vi "addEdge.vi"(0 "reference":refnum<class "NoteNode.lvclass">, 1 "egde":refnum<class "AbstractEdge.lvclass">, 2 "p1":T1 {"y" format="%.2f"; "x" format="%.2f"}, 3 "p2":T1 {"y" format="%.2f"; "x" format="%.2f"}, 5 "error in (no error)":errorcluster) -> (14 "reference out":refnum<class "NoteNode.lvclass">, 15 "edgeHasEndNode":bool, 19 "error out":errorcluster)   [LabVIEW 2012, in "NoteNode.lvclass"]
doc: "public boolean addEdge(Edge e, Point2D p1, Point2D p2)"
uses:
  <resource>/Framework/Providers/Open_GDS/UML/NoteNode_class/NoteNode.lvclass
  <resource>/Framework/Providers/Open_GDS/UML/AbstractEdge_class/AbstractEdge.lvclass
  <resource>/Framework/Providers/Open_GDS/UML/General/Point/Point Point2D.ctl
  <resource>/Framework/Providers/Open_GDS/UML/RectangularNode_class/RectangularNode.lvclass
  <resource>/Framework/Providers/Open_GDS/UML/PointNode_class/PointNode.lvclass
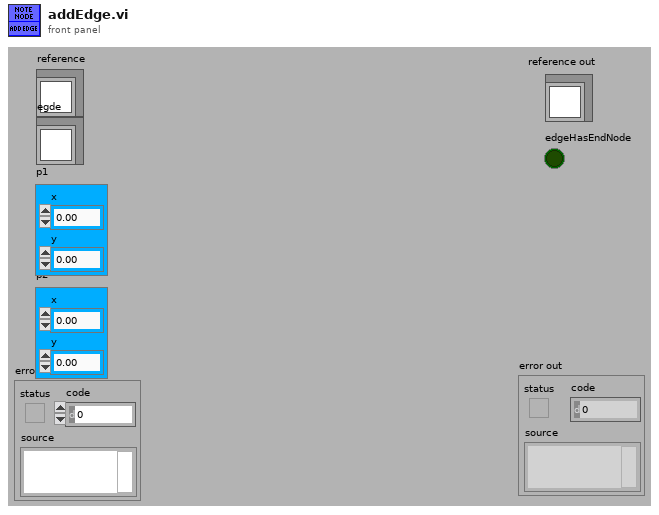
[diagram p1: front panel]
types:
  T1 = typedef "Point Point2D.ctl" = cluster{"x":dbl, "y":dbl}
  T2 = typedef "NoteNode.lvclass/ObjectAttributes.ctl" = cluster{"Base class":T3, "DEFAULT_WIDTH":i32, "DEFAULT_HEIGHT":i32, "DEFAULT_COLOR":u32, "FOLD_X":i32, "FOLD_Y":i32, "color":u32, "text":refnum<class "MultiLineString.lvclass">, "pointNodes":refnum<class "AbstractNode.lvclass">[]}
  T3 = typedef "RectangularNode.lvclass/ObjectAttributes.ctl" = cluster{"Base class":T4, "bounds":T5}
  T4 = typedef "AbstractNode.lvclass/ObjectAttributes.ctl" = cluster{"parent":refnum<class "AbstractNode.lvclass">, "children":refnum<class "AbstractNode.lvclass">[], "Hidden":bool}
  T5 = typedef "Rectangle Rectangle2D.ctl" = cluster{"x":dbl, "y":dbl, "width":dbl, "height":dbl}
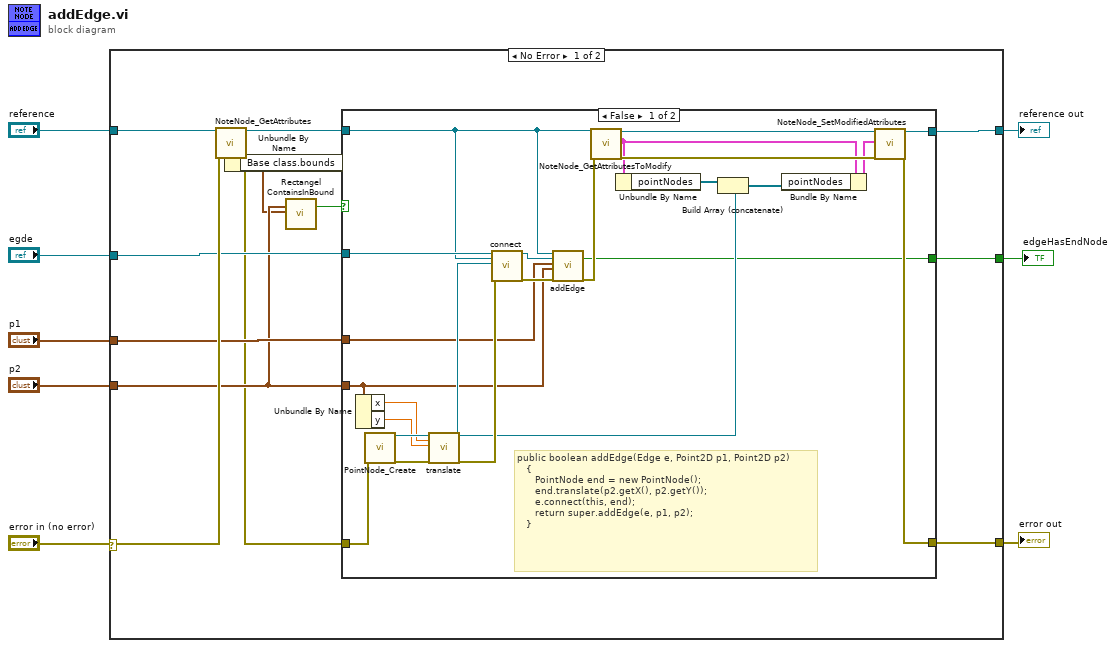
[diagram p0: block diagram]
diagram:
  n1 = case shown="No Error" "error in (no error)" {
    selector: "error in (no error)" -> [w18 w47]
    tunnel: "reference" -> [w21 w48]
    tunnel: [w20 w47] -> w7
    tunnel: [w19 w48] -> w6
    tunnel: "egde" -> [w17 _]
    tunnel: "p1" -> [w16 _]
    tunnel: "p2" -> [w15 _]
    tunnel: [w9 _] -> w1
    frame No Error {
      n2 = call <resource>:"NoteNode_GetAttributes.vi"("reference in"=w21, "error in (no error)"=w18) -> ("reference out"=w14:refnum<class "NoteNode.lvclass">, "Attributes"=w12:T2, "error out"=w13:errorcluster)  [unwired: 15 out]
      n3 = Unbundle By Name(w12) -> ("Base class.bounds"=w11:T5)
      n4 = call <resource>:"Rectangel ContainsInBound.vi"("point2D"=w15, "bounds"=w11) -> ("contains"=w10:bool)  [unwired: 2 in, 15 out]
      n5 = case shown="False" w10 {
        tunnel: w17 -> [w44 _]
        tunnel: w16 -> [w25 _]
        tunnel: [w36 w46] -> w19
        tunnel: [w35 w45] -> w20
        tunnel: w14 -> [w28 w46]
        tunnel: w13 -> [w29 w45]
        tunnel: w15 -> [w24 _]
        tunnel: [w22 _] -> w9
        frame False {
          # "public boolean addEdge(Edge e, Point2D p1, Point2D p2)\n   {\n      PointNode end = new PointNode();\n      end.translate(p2.getX(), p2.getY());\n      e.connect(this, end);\n      return super.addEdge(e, p1, p2);\n   }"
          n6 = Unbundle By Name(w24) -> ("x"=w41:dbl, "y"=w40:dbl)
          n7 = call <resource>:"PointNode_Create.vi"("error in (no error)"=w29) -> ("reference out"=w43:refnum<class "PointNode.lvclass">, "error out"=w42:errorcluster)  [unwired: 2 in, 15 out]
          n8 = call-dynamic "translate.vi"("reference"=w43, "dx"=w41, "dy"=w40, "error in (no error)"=w42) -> ("reference out"=w30:refnum<class "PointNode.lvclass">, "error out"=w39:errorcluster)  [unwired: 14 in]
          n9 = call-dynamic "connect.vi"("reference"=w44, "startNode"=w28, "endNode"=w30, "error in (no error)"=w39) -> ("reference out"=w26:refnum<class "AbstractEdge.lvclass">, "error out"=w27:errorcluster)  [unwired: 14 in]
          n10 = call-parent "addEdge.vi"("reference"=w28, "egde"=w26, "p1"=w25, "p2"=w24, "error in (no error)"=w27) -> ("edgeHasEndNode"=w22:bool, "error out"=w23:errorcluster)  [unwired: 12 in, 1 out]
          n11 = call <resource>:"NoteNode_GetAttributesToModify.vi"("reference in"=w28, "error in (no error)"=w23) -> ("reference out"=w38:refnum<class "NoteNode.lvclass">, "Attributes"=w34:T2, "error out"=w37:errorcluster)  [unwired: 1 in, 14 out]
          n12 = Unbundle By Name(w34) -> ("pointNodes"=w32:refnum<class "AbstractNode.lvclass">[])
          n13 = Build Array (concatenate)(w32, w30) -> (w31:refnum<class "AbstractNode.lvclass">[])
          n14 = Bundle By Name(cluster=w34, "pointNodes"=w31) -> (w33:T2)
          n15 = call <resource>:"NoteNode_SetModifiedAttributes.vi"("reference in"=w38, "Attributes"=w33, "error in (no error)"=w37) -> ("reference out"=w36:refnum<class "NoteNode.lvclass">, "error out"=w35:errorcluster)  [unwired: 3 in, 12 out]
        }
        frame True {
        }
      }
    }
    frame Error {
    }
  }
  "reference out" <- w6
  "error out" <- w7
  "edgeHasEndNode" <- w1
